vi "ETAS_Driver_1.0.2.vi"(6 "Counter In":dbl format="%#_13g", 7 "IP Address":string, 8 "Loop In":i32, 9 "error In":errorcluster, 10 "Reference In":refnum<k24>, 11 "Etas Connect":bool) -> (0 "Loop Out":i32, 1 "error out":errorcluster, 2 "Reference Out":refnum<k24>, 3 "ETAS Out":dbl[](array[numeric]), 4 "Counter Out":dbl format="%#_13g")   [LabVIEW 2014]
uses:
  C:/Users/JonnyS/Desktop/OMEGA_14/Windows/SubVIs Win/ETASdigital.dll
  ETASdigital.dll
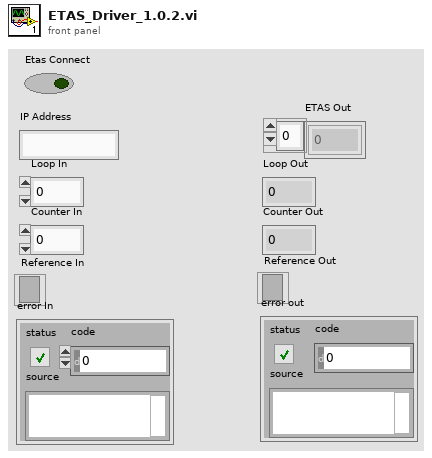
[diagram p1: front panel]
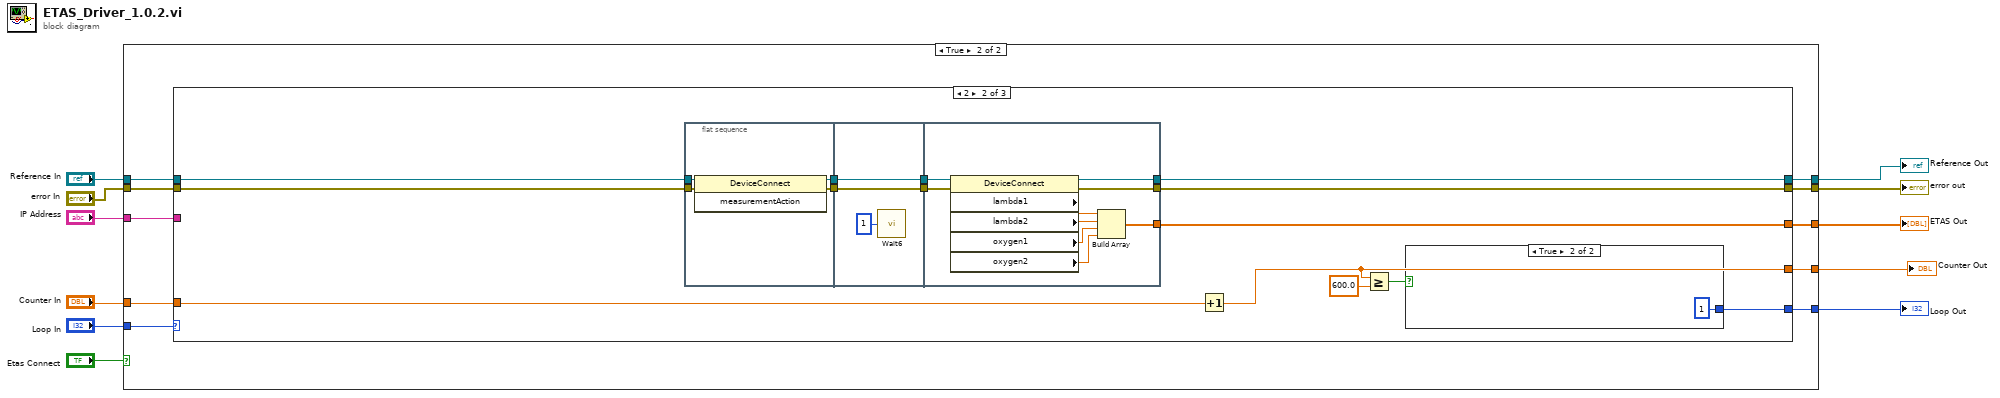
[diagram p0: block diagram]
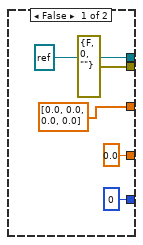
[diagram p2: hidden frame]
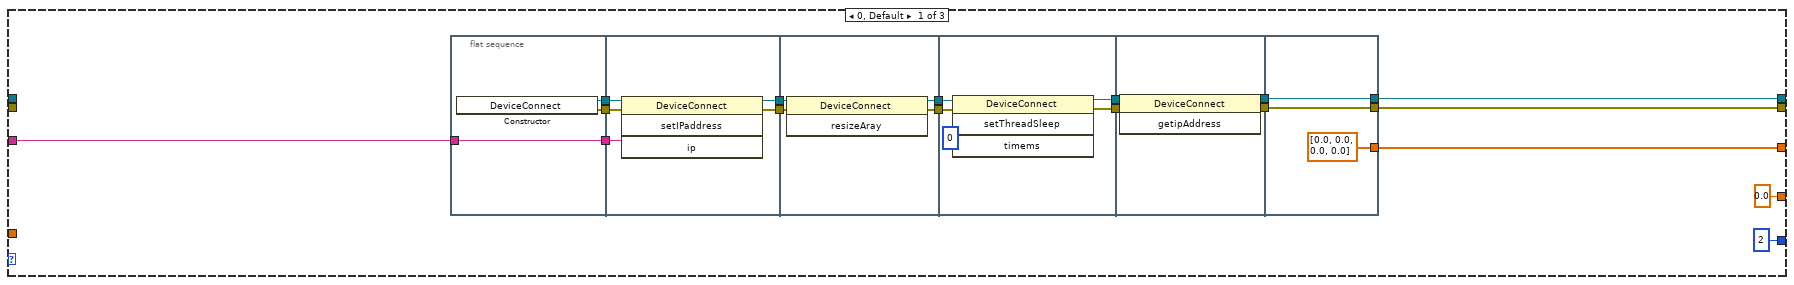
[diagram p3: hidden frame]
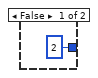
[diagram p4: hidden frame]
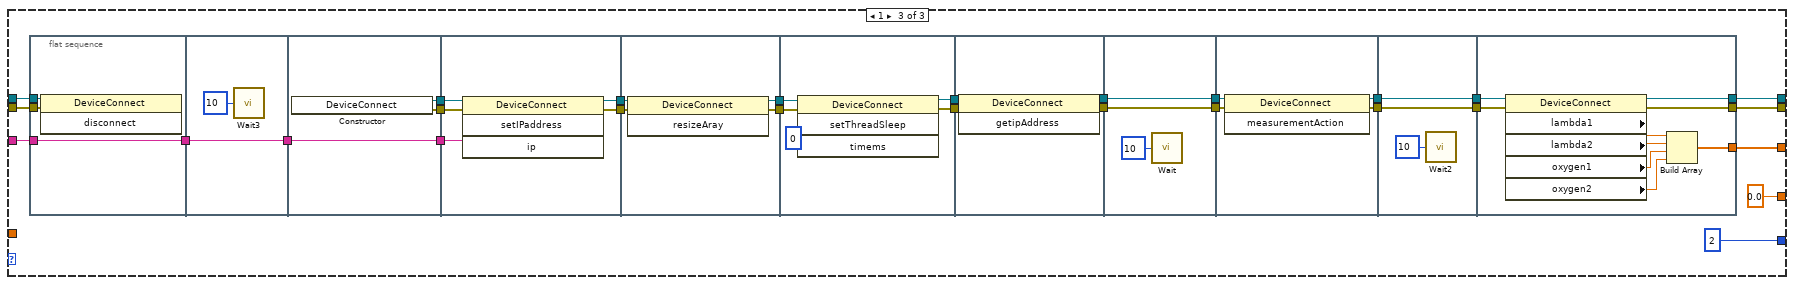
[diagram p5: hidden frame]
diagram:
  n1 = case shown="True" "Etas Connect" {
    tunnel: "Reference In" -> [_ w26]
    tunnel: "error In" -> [_ w25]
    tunnel: [0.0 ("x") w24] -> w8
    tunnel: [0 ("Loop Out") w23] -> w7
    tunnel: [dbl[] [0.0, 0.0, 0.0, 0.0] w22] -> w6
    tunnel: [refnum<k24> refnum ("new reference") w21] -> w5
    tunnel: [errorcluster {"status"=FALSE, "code"=0, "source"=""} ("error out") w20] -> w4
    tunnel: "Counter In" -> [_ w19]
    tunnel: "Loop In" -> [_ w18]
    tunnel: "IP Address" -> [_ w17]
    frame False {
    }
    frame True {
      n2 = case shown="2" w18 {
        tunnel: [w33 w77 w110] -> w21
        tunnel: [w32 w76 w109] -> w20
        tunnel: [w31 w75 w108] -> w22
        tunnel: [2 ("Loop Out") w74 2 ("Loop Out")] -> w23
        tunnel: w26 -> [_ w69 w106]
        tunnel: w25 -> [_ w68 w105]
        tunnel: [0.0 ("x") w71 0.0 ("x")] -> w24
        tunnel: w19 -> [_ w70 _]
        tunnel: w17 -> [w27 _ w103]
        frame 0, Default {
          n3 = flat-sequence {
            tunnel: [w46] -> w43
            tunnel: [w45] -> w42
            tunnel: [w44] -> w28
            tunnel: w27 -> [w44]
            tunnel: w43 -> [w51]
            tunnel: w42 -> [w50]
            tunnel: [w49] -> w41
            tunnel: [w48] -> w40
            tunnel: w28 -> [w47]
            tunnel: w41 -> [w55]
            tunnel: w40 -> [w54]
            tunnel: [w53] -> w39
            tunnel: [w52] -> w38
            tunnel: w39 -> [w59]
            tunnel: w38 -> [w58]
            tunnel: [w57] -> w37
            tunnel: [w56] -> w36
            tunnel: w37 -> [w64]
            tunnel: w36 -> [w63]
            tunnel: [w62] -> w35
            tunnel: [w61] -> w34
            tunnel: [w67] -> w33
            tunnel: w35 -> [w67]
            tunnel: [w66] -> w32
            tunnel: w34 -> [w66]
            tunnel: [dbl[] [0.0, 0.0, 0.0, 0.0]] -> w31
            frame #0 {
              n4 = constructor class="DeviceConnect"() -> (reference out=w46:refnum<k24>, error out=w45:errorcluster)  [unwired: 3 in, 1 out]
            }
            frame #1 {
              n5 = invoke class="DeviceConnect" method="setIPaddress"(reference=w51, error in=w50, "ip"=w47) -> (reference out=w49:refnum<k24>, error out=w48:errorcluster)  [unwired: 1 in, 2 out]
            }
            frame #2 {
              n6 = invoke class="DeviceConnect" method="resizeAray"(reference=w55, error in=w54) -> (reference out=w53:refnum<k24>, error out=w52:errorcluster)  [unwired: 1 in, 1 out]
            }
            frame #3 {
              n7 = invoke class="DeviceConnect" method="setThreadSleep"(reference=w59, error in=w58, "timems"=0) -> (reference out=w57:refnum<k24>, error out=w56:errorcluster)  [unwired: 1 in, 2 out]
            }
            frame #4 {
              n8 = invoke class="DeviceConnect" method="getipAddress"(reference=w64, error in=w63) -> (reference out=w62:refnum<k24>, error out=w61:errorcluster)  [unwired: 1 in, 1 out]
            }
            frame #5 {
            }
          }
        }
        frame 2 {
          n9 = flat-sequence {
            tunnel: [w87] -> w81
            tunnel: [w86] -> w80
            tunnel: w69 -> [w85]
            tunnel: w68 -> [w84]
            tunnel: w81 -> [w90]
            tunnel: w80 -> [w89]
            tunnel: [w90] -> w79
            tunnel: [w89] -> w78
            tunnel: w79 -> [w99]
            tunnel: w78 -> [w94]
            tunnel: [w93] -> w77
            tunnel: [w92] -> w76
            tunnel: [w91] -> w75
            frame #0 {
              n10 = invoke class="DeviceConnect" method="measurementAction"(reference=w85, error in=w84) -> (reference out=w87:refnum<k24>, error out=w86:errorcluster)  [unwired: 1 in, 1 out]
            }
            frame #1 {
              n11 = call "Wait6"("Count(mSec)"=u32 1) -> ()  [unwired: 1 out]
            }
            frame #2 {
              n12 = property class="DeviceConnect"(reference=w99, error in=w94) -> (reference out=w93:refnum<k24>, error out=w92:errorcluster, "lambda1"=w98:dbl, "lambda2"=w97:dbl, "oxygen1"=w96:dbl, "oxygen2"=w95:dbl)
              n13 = Build Array(w98, w97, w96, w95) -> (w91:dbl[])
            }
          }
          n14 = Increment(x=w70) -> (x+1=w71:dbl)
          n15 = Greater Or Equal?(x=w71, y=600.0) -> (x >= y?=w73:bool)
          n16 = case shown="True" w73 {
            tunnel: [2 ("Loop Out") 1 ("Loop Out")] -> w74
            frame False {
            }
            frame True {
            }
          }
        }
        frame 1 {
          n17 = flat-sequence {
            tunnel: w106 -> [w129]
            tunnel: w105 -> [w128]
            tunnel: w103 -> [w127]
            tunnel: [w127] -> w100
            tunnel: [w130] -> w101
            tunnel: w100 -> [w130]
            tunnel: [w134] -> w126
            tunnel: [w133] -> w125
            tunnel: [w132] -> w102
            tunnel: w101 -> [w132]
            tunnel: w126 -> [w139]
            tunnel: w125 -> [w138]
            tunnel: [w137] -> w124
            tunnel: [w136] -> w123
            tunnel: w102 -> [w135]
            tunnel: w124 -> [w143]
            tunnel: w123 -> [w142]
            tunnel: [w141] -> w122
            tunnel: [w140] -> w121
            tunnel: w122 -> [w147]
            tunnel: w121 -> [w146]
            tunnel: [w145] -> w120
            tunnel: [w144] -> w119
            tunnel: w120 -> [w152]
            tunnel: w119 -> [w151]
            tunnel: [w150] -> w118
            tunnel: [w149] -> w117
            tunnel: w118 -> [w155]
            tunnel: w117 -> [w154]
            tunnel: [w155] -> w116
            tunnel: [w154] -> w115
            tunnel: w116 -> [w159]
            tunnel: w115 -> [w158]
            tunnel: [w157] -> w114
            tunnel: [w156] -> w113
            tunnel: w114 -> [w162]
            tunnel: w113 -> [w161]
            tunnel: [w162] -> w112
            tunnel: [w161] -> w111
            tunnel: w112 -> [w171]
            tunnel: w111 -> [w166]
            tunnel: [w165] -> w110
            tunnel: [w164] -> w109
            tunnel: [w163] -> w108
            frame #0 {
              n18 = invoke class="DeviceConnect" method="disconnect"(reference=w129, error in=w128) -> ()  [unwired: 1 in, 3 out]
            }
            frame #1 {
              n19 = call "Wait3"("Count(mSec)"=u32 10) -> ()  [unwired: 1 out]
            }
            frame #2 {
              n20 = constructor class="DeviceConnect"() -> (reference out=w134:refnum<k24>, error out=w133:errorcluster)  [unwired: 3 in, 1 out]
            }
            frame #3 {
              n21 = invoke class="DeviceConnect" method="setIPaddress"(reference=w139, error in=w138, "ip"=w135) -> (reference out=w137:refnum<k24>, error out=w136:errorcluster)  [unwired: 1 in, 2 out]
            }
            frame #4 {
              n22 = invoke class="DeviceConnect" method="resizeAray"(reference=w143, error in=w142) -> (reference out=w141:refnum<k24>, error out=w140:errorcluster)  [unwired: 1 in, 1 out]
            }
            frame #5 {
              n23 = invoke class="DeviceConnect" method="setThreadSleep"(reference=w147, error in=w146, "timems"=0) -> (reference out=w145:refnum<k24>, error out=w144:errorcluster)  [unwired: 1 in, 2 out]
            }
            frame #6 {
              n24 = invoke class="DeviceConnect" method="getipAddress"(reference=w152, error in=w151) -> (reference out=w150:refnum<k24>, error out=w149:errorcluster)  [unwired: 1 in, 1 out]
            }
            frame #7 {
              n25 = call "Wait"("Count(mSec)"=u32 10) -> ()  [unwired: 1 out]
            }
            frame #8 {
              n26 = invoke class="DeviceConnect" method="measurementAction"(reference=w159, error in=w158) -> (reference out=w157:refnum<k24>, error out=w156:errorcluster)  [unwired: 1 in, 1 out]
            }
            frame #9 {
              n27 = call "Wait2"("Count(mSec)"=u32 10) -> ()  [unwired: 1 out]
            }
            frame #10 {
              n28 = property class="DeviceConnect"(reference=w171, error in=w166) -> (reference out=w165:refnum<k24>, error out=w164:errorcluster, "lambda1"=w170:dbl, "lambda2"=w169:dbl, "oxygen1"=w168:dbl, "oxygen2"=w167:dbl)
              n29 = Build Array(w170, w169, w168, w167) -> (w163:dbl[])
            }
          }
        }
      }
    }
  }
  "ETAS Out" <- w6
  "Loop Out" <- w7
  "Reference Out" <- w5
  "error out" <- w4
  "Counter Out" <- w8
